vi "Insert Namespace.vi"(4 "Test File Version Number":string, 8 "error in (no error)":errorcluster, 9 "Linked List ID":string, 10 "Name":string, 11 "Test Executive in":refnum<class "Test Executive.lvclass">) -> (0 "error out":errorcluster, 1 "Replaced?":bool, 3 "Test Executive out":refnum<class "Test Executive.lvclass">, 5 "Unique ID out":string)   [LabVIEW 2020, in "Test Executive.lvlib" / "Test Executive.lvclass"]
uses:
  <vilib>/gpm_packages/@cs/test-executive/Source/Test Executive/TestExecutive/Test Executive.lvclass
  <vilib>/gpm_packages/@cs/test-executive/Source/Test Executive/Name Space/Name Space.lvclass
  <vilib>/gpm_packages/@cs/test-executive/Source/Test Executive/TestExecutive/Test Executive.lvclass/Test Executive.ctl
  430d272f-7f9c-469f-be8b-e7711a474498.vi
  <vilib>/gpm_packages/@cs/linked-list/Source/Linked List/ILinkedList/ILinked List.lvclass
  <vilib>/gpm_packages/@cs/linked-list/Source/Linked List/Linked List Ref/Linked List Ref.lvclass
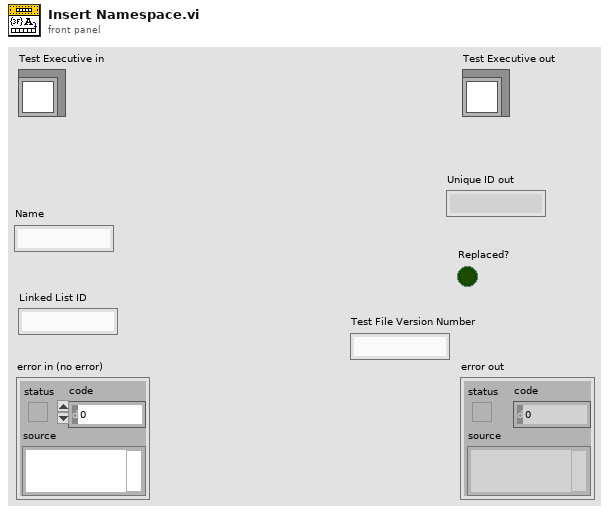
[diagram p1: front panel]
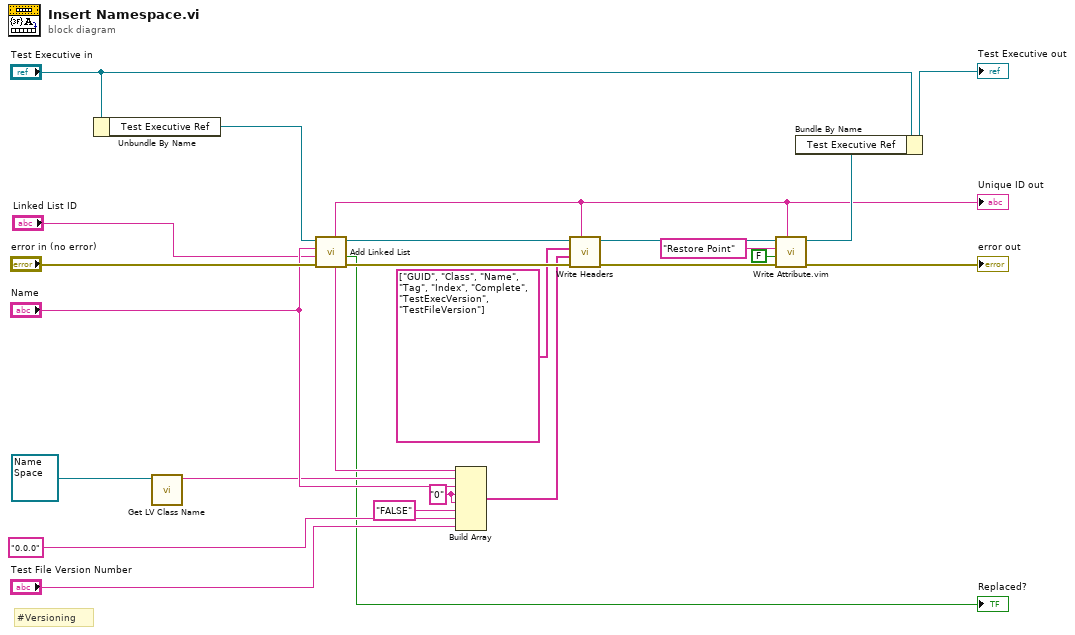
[diagram p0: block diagram]
diagram:
  w9 = "0" ("element")
  # "#Versioning"
  n1 = Unbundle By Name("Test Executive in") -> ("Test Executive Ref"=w24:refnum<data-value>)
  n2 = call <vilib>:"Get LV Class Name.vi"("object"=refnum<class "Name Space.lvclass"> refnum ("Test Executive.lvlib:Name Space.lvclass")) -> ("class name"=w11:string)  [unwired: 9 in, 1 out]
  n3 = call <vilib>:"Add Linked List.vi"("error in (no error)"="error in (no error)", "Linked List ID"="Linked List ID", "Name"="Name", "Linked List Ref"=w24) -> ("error out"=w22:errorcluster, "Replaced?"=→"Replaced?":bool, "Linked List Ref out"=w23:refnum<data-value>, "Linked List ID out"=w7:string)  [unwired: 4 in]
  "Unique ID out" <- w7
  n4 = Build Array(w7, w11, "Name", w9, w9, "FALSE" ("element"), "0.0.0" ("Test Executive Version Number"), "Test File Version Number") -> (w20:string[])
  n5 = call <vilib>:"Write Headers.vi"("Linked List ID"=w7, "error in (no error)"=w22, "Header Values"=w20, "Header Names"=string[] ["GUID", "Class", "Name", "Tag", "Index", "Complete", "TestExecVersion", "TestFileVersion"], "Linked List Ref"=w23) -> ("error out"=w5:errorcluster, "Linked List Ref out"=w6:refnum<data-value>)  [unwired: 5 in]
  n6 = call "Write Attribute.vim"("Linked List ID"=w7, "error in (no error)"=w5, "Attribute"=FALSE, "Attribute Name"="Restore Point", "Linked List Ref"=w6) -> ("error out"=→"error out":errorcluster, "Linked List Ref out"=w17:refnum<data-value>)  [unwired: 3 in, 2 out]
  n7 = Bundle By Name(cluster="Test Executive in", "Test Executive Ref"=w17) -> (→"Test Executive out":refnum<class "Test Executive.lvclass">)
